vi "Handle SUBSCRIBED.vi"(0 "reference":refnum<class "WAMP Client.lvclass">, 5 "WAMP Message":T1 {"Message Codes" items=["HELLO"=1, "WELCOME"=2, "ABORT"=3, "GOODBYE"=6, "ERROR"=8, "PUBLISH"=16, "PUBLISHED"=17, "SUBSCRIBE"=32, "SUBSCRIBED"=33, "UNSUBSCRIBE"=34, "UNSUBSCRIBED"=35, "EVENT"=36, "CALL"=48, "RESULT"=59, "REGISTER"=64, "REGISTERED"=65, "UNREGISTER"=66, "UNREGISTERED"=67, "INVOCATION"=68, "YIELD"=70]}, 9 "Message Loop data (in)":T3, 11 "error in (no error)":errorcluster) -> (4 "reference out":refnum<class "WAMP Client.lvclass">, 10 "Message Loop Data (out)":T3, 15 "error out":errorcluster)   [LabVIEW 2020, in "wamplv.lvlib" / "WAMP Client.lvclass"]
uses:
  WAMP Client.lvclass
  TypeDef/Message Loop Data.ctl
  TypeDef/REGISTER Request Data.ctl
  TypeDef/Success or error.ctl
  API/TypeDefs/Combined error.ctl
  API/TypeDefs/WAMP error.ctl
  TypeDef/Publish Requests Map.ctl
  TypeDef/PUBLISH Request Data.ctl
  TypeDef/PUBLISH result.ctl
  TypeDef/Endpoint Data.ctl
  TypeDef/CALL Request Map.ctl
  TypeDef/CALL Request Data.ctl
  API/TypeDefs/RESULT payload.ctl
  TypeDef/SUBSCRIBE Requests Map.ctl
  TypeDef/SUBSCRIBE Request Data.ctl
  TypeDef/Subscribe Result.ctl
  TypeDef/EVENT payload.ctl
  TypeDef/Subscriptions Map.ctl
  TypeDef/Subscription Details.ctl
  TypeDef/Unsubscribe Requests Map.ctl
  TypeDef/UNSUBSCRIBE Request Data.ctl
  TypeDef/UNSUBSCRIBE Result.ctl
  TypeDef/Unregister requests map.ctl
  TypeDef/Unregister request.ctl
  TypeDef/WAMP Received Message.ctl
  TypeDef/WAMP Message Codes.ctl
  4df5dd5f-e550-40b2-bd6e-53c88ea5040d.vi
  WAMP Client.lvclass/WAMP Client.ctl
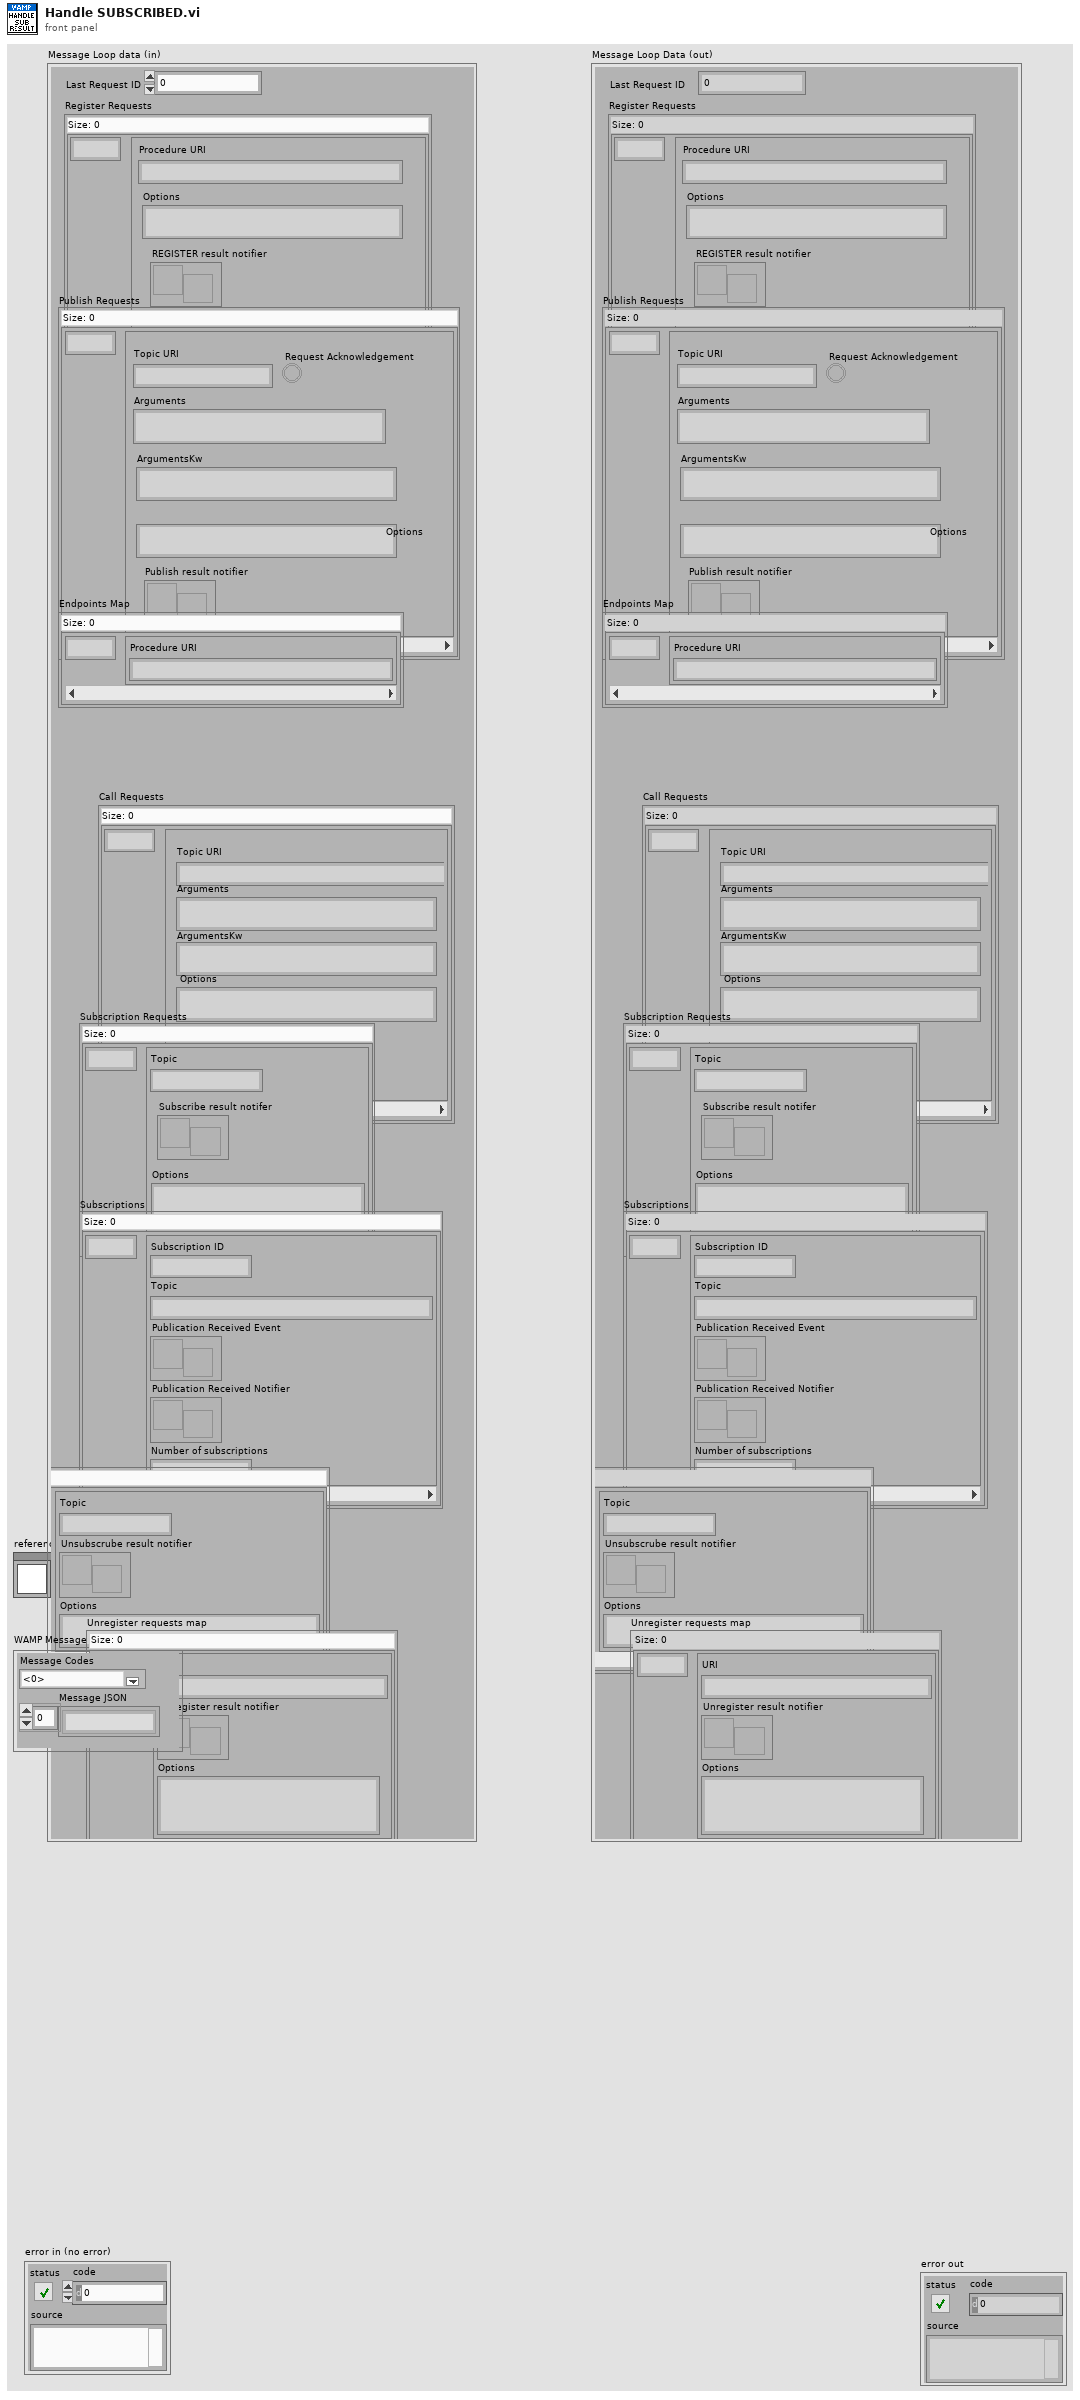
[diagram p1: front panel]
types:
  T1 = typedef "wamplv.lvlib/WAMP Client.lvclass/WAMP Received Message.ctl" = cluster{"Message JSON":string[], "Message Codes":T2}
  T2 = typedef "wamplv.lvlib/WAMP Client.lvclass/WAMP Message Codes.ctl" = u16
  T3 = typedef "wamplv.lvlib/WAMP Client.lvclass/Message Loop Data.ctl" = cluster{"Last Request ID":u64, "Register Requests":map{u64, T4}, "Publish Requests":T5, "Endpoints Map":map{u64, T7}, "Call Requests":T8, "Subscription Requests":T10, "Subscriptions":T12, "Unsubscribe Requests":T14, "Random Request IDs":u64[], "Unregister requests map":T16}
  T4 = typedef "wamplv.lvlib/WAMP Client.lvclass/REGISTER Request Data.ctl" = cluster{"Procedure URI":string, "Options":string, "REGISTER result notifier":refnum<notifier>}
  T5 = typedef "wamplv.lvlib/WAMP Client.lvclass/Publish Requests Map.ctl" = map{u64, T6}
  T6 = typedef "wamplv.lvlib/WAMP Client.lvclass/PUBLISH Request Data.ctl" = cluster{"Topic URI":string, "Arguments":string, "ArgumentsKw":string, "Request Acknowledgement":bool, "Options":string, "Publish result notifier":refnum<notifier>}
  T7 = typedef "wamplv.lvlib/WAMP Client.lvclass/Endpoint Data.ctl" = cluster{"Procedure URI":string}
  T8 = typedef "wamplv.lvlib/WAMP Client.lvclass/CALL Request Map.ctl" = map{u64, T9}
  T9 = typedef "wamplv.lvlib/WAMP Client.lvclass/CALL Request Data.ctl" = cluster{"Topic URI":string, "Arguments":string, "ArgumentsKw":string, "Options":string, "Call result":refnum<notifier>}
  T10 = typedef "wamplv.lvlib/WAMP Client.lvclass/SUBSCRIBE Requests Map.ctl" = map{u64, T11}
  T11 = typedef "wamplv.lvlib/WAMP Client.lvclass/SUBSCRIBE Request Data.ctl" = cluster{"Topic":string, "Subscribe result notifer":refnum<notifier>, "Options":string}
  T12 = typedef "wamplv.lvlib/WAMP Client.lvclass/Subscriptions Map.ctl" = map{u64, T13}
  T13 = typedef "wamplv.lvlib/WAMP Client.lvclass/Subscription Details.ctl" = cluster{"Subscription ID":u64, "Topic":string, "Publication Received Event":refnum<user-event>, "Publication Received Notifier":refnum<notifier>, "Number of subscriptions":u64}
  T14 = typedef "wamplv.lvlib/WAMP Client.lvclass/Unsubscribe Requests Map.ctl" = map{u64, T15}
  T15 = typedef "wamplv.lvlib/WAMP Client.lvclass/UNSUBSCRIBE Request Data.ctl" = cluster{"Topic":string, "Unsubscrube result notifier":refnum<notifier>, "Options":string}
  T16 = typedef "wamplv.lvlib/WAMP Client.lvclass/Unregister requests map.ctl" = map{u64, T17}
  T17 = typedef "wamplv.lvlib/WAMP Client.lvclass/Unregister request.ctl" = cluster{"URI":string, "Unregister result notifier":refnum<notifier>, "Options":string}
  T18 = typedef "wamplv.lvlib/WAMP Client.lvclass/Subscribe Result.ctl" = cluster{"Success?":bool, "Publication Received Event":refnum<user-event>, "Publication Received Notifier":refnum<notifier>, "Combined Error":T19}
  T19 = typedef "wamplv.lvlib/WAMP Client.lvclass/Combined error.ctl" = cluster{"Error?":bool, "WAMP Error":T20, "Error":errorcluster}
  T20 = typedef "wamplv.lvlib/WAMP Client.lvclass/WAMP error.ctl" = cluster{"Details":string, "ArgumentKw Payload":string, "Error?":bool, "Error URI":string, "Arguments Payload":string}
  T21 = typedef "wamplv.lvlib/WAMP Client.lvclass/EVENT payload.ctl" = cluster{"Arguments Payload":string, "ArgumentKw Payload":string, "Topic":string}
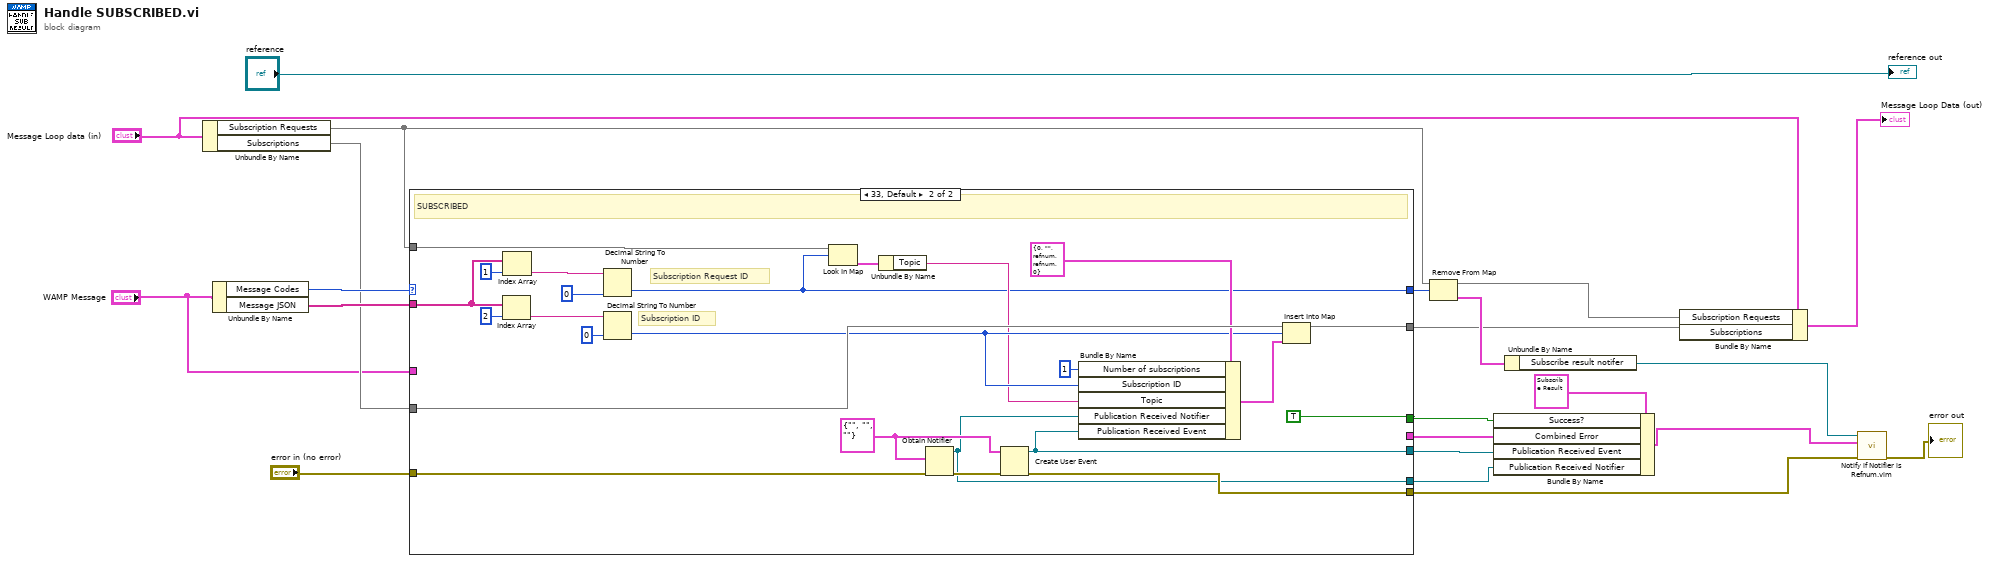
[diagram p0: block diagram]
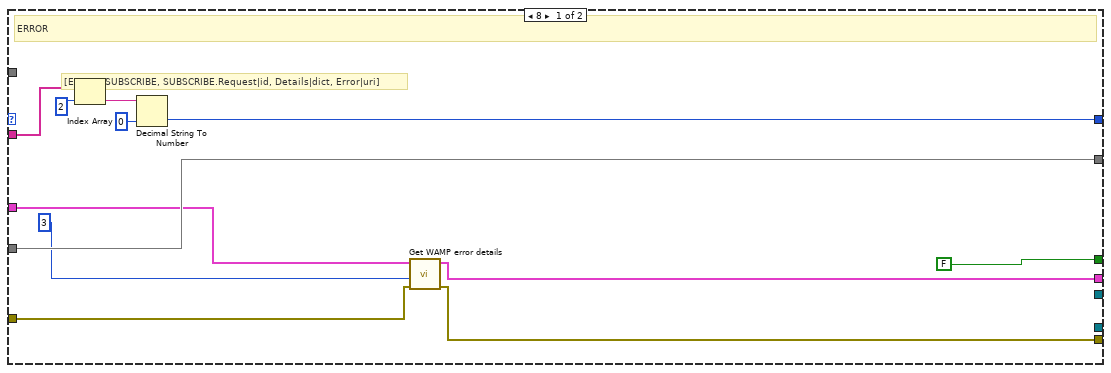
[diagram p2: hidden frame]
diagram:
  n1 = Unbundle By Name("Message Loop data (in)") -> ("Subscription Requests"=w13:T10, "Subscriptions"=w12:T12)
  n2 = Unbundle By Name("WAMP Message") -> ("Message Codes"=w18:T2, "Message JSON"=w17:string[])
  n3 = case shown="33, Default" w18 {
    tunnel: w17 -> [w32 w55]
    tunnel: [w30 w36] -> w16
    tunnel: "error in (no error)" -> [w23 w41]
    tunnel: [w24 w42] -> w3
    tunnel: [FALSE ("Success?") TRUE ("Success?")] -> w20
    tunnel: w12 -> [w29 w50]
    tunnel: w13 -> [_ w46]
    tunnel: [w29 w43] -> w8
    tunnel: [_ w38] -> w14
    tunnel: [w25 _] -> w7
    tunnel: "WAMP Message" -> [w26 _]
    tunnel: [_ w37] -> w1
    frame 8 {
      # "[ERROR, SUBSCRIBE, SUBSCRIBE.Request|id, Details|dict, Error|uri]"
      # "ERROR"
      n4 = Index Array(array=w32, index=2) -> (element=w33:string)
      n5 = Decimal String To Number(string=w33, default (0L)=u64 0 ("default (0 I32)")) -> (number=w30:u64)  [unwired: 1 in, 1 out]
      n6 = call "Get WAMP error details.vi"("error in (no error)"=w23, "Details Index"=u32 3, "WAMP Message"=w26) -> ("error out"=w24:errorcluster, "Combined Error"=w25:T19)  [unwired: 6 in, 1 out]
    }
    frame 33, Default {
      w39 = T21 {"Arguments Payload"="", "ArgumentKw Payload"="", "Topic"=""} ("Cluster")
      # "Subscription Request ID"
      # "Subscription ID"
      # "SUBSCRIBED"
      n7 = Index Array(array=w55, index=2) -> (element=w57:string)
      n8 = Index Array(array=w55, index=1) -> (element=w53:string)
      n9 = Decimal String To Number(string=w53, default (0L)=u64 0) -> (number=w36:u64)  [unwired: 1 in, 1 out]
      n10 = Decimal String To Number(string=w57, default (0L)=u64 0) -> (number=w48:u64)  [unwired: 1 in, 1 out]
      n11 = Look In Map(map=w46, key=w36) -> (value=w45:T11)  [unwired: 1 in, 1 out]
      n12 = Unbundle By Name(w45) -> ("Topic"=w44:string)
      n13 = Obtain Notifier(notification data type=w39, error in (no error)=w41) -> (notifier out=w37:refnum<notifier>, error out=w40:errorcluster)  [unwired: 2 in, 1 out]
      n14 = Create User Event(user event datatype=w39, error in=w40) -> (user event=w38:refnum<user-event>, error out=w42:errorcluster)
      n15 = Bundle By Name(cluster=T13 {"Subscription ID"=0, "Topic"="", "Publication Received Event"=refnum, "Publication Received Notifier"=refnum, "Number of subscriptions"=0} ("Cluster"), "Number of subscriptions"=u64 1, "Subscription ID"=w48, "Topic"=w44, "Publication Received Notifier"=w37, "Publication Received Event"=w38) -> (w47:T13)
      n16 = Insert Into Map(map in=w50, key=w48, value=w47) -> (map out=w43:T12)  [unwired: 2 out]
    }
  }
  n17 = Remove From Map(10:w16, 11:w13) -> (1:w15:T11, 3:w11:T10)  [unwired: 1 out]
  n18 = Bundle By Name(cluster=T18 {"Success?"=FALSE, "Publication Received Event"=refnum, "Publication Received Notifier"=refnum, "Combined Error"={"Error?"=FALSE, "WAMP Error"={"Details"="", "ArgumentKw Payload"="{}", "Error?"=FALSE, "Error URI"="", "Arguments Payload"=""}, "Error"={"status"=FALSE, "code"=0, "source"=""}}} ("event data"), "Success?"=w20, "Combined Error"=w7, "Publication Received Event"=w14, "Publication Received Notifier"=w1) -> (w4:T18)
  n19 = Unbundle By Name(w15) -> ("Subscribe result notifer"=w5:refnum<notifier>)
  n20 = Bundle By Name(cluster="Message Loop data (in)", "Subscription Requests"=w11, "Subscriptions"=w8) -> (→"Message Loop Data (out)":T3)
  n21 = call "Notify if Notifier is Refnum.vim"("error in (no error)"=w3, "RESULT Payload"=w4, "Notifier in"=w5) -> ("error out"=→"error out":errorcluster)  [unwired: 8 in]
  "reference out" <- "reference"
